vi "颖洁的新生日志_main.vi"() -> ()   [LabVIEW 2011]
panel:
  in  "圈存机":bool
  out "等级":i32=1000
  out "leave":bool
  in  "退出？":bool
  in  "退出游戏":bool
  out "开心值":dbl(slide) scale=0.0..500.0
  out "当前开心值":i32=1000
  out "提示":string
  in  "银行":bool
  out "存款":i32
  in  "云杉轩":bool
  in  "海棠轩":bool
  out "天数":i32
  out "余额":i32
  in  "辛夷阁":bool
  in  "枕雨楼":bool
  in  "库存":i32[](listbox)
  in  "卖出数量":i32 min=0 step=1
  in  "买入数量":i32 min=0 step=1
  in  "卖出":bool
  in  "买入":bool
  in  "商品价格":i32[](listbox)
  out "物品存在索引":i32[](array[numeric])
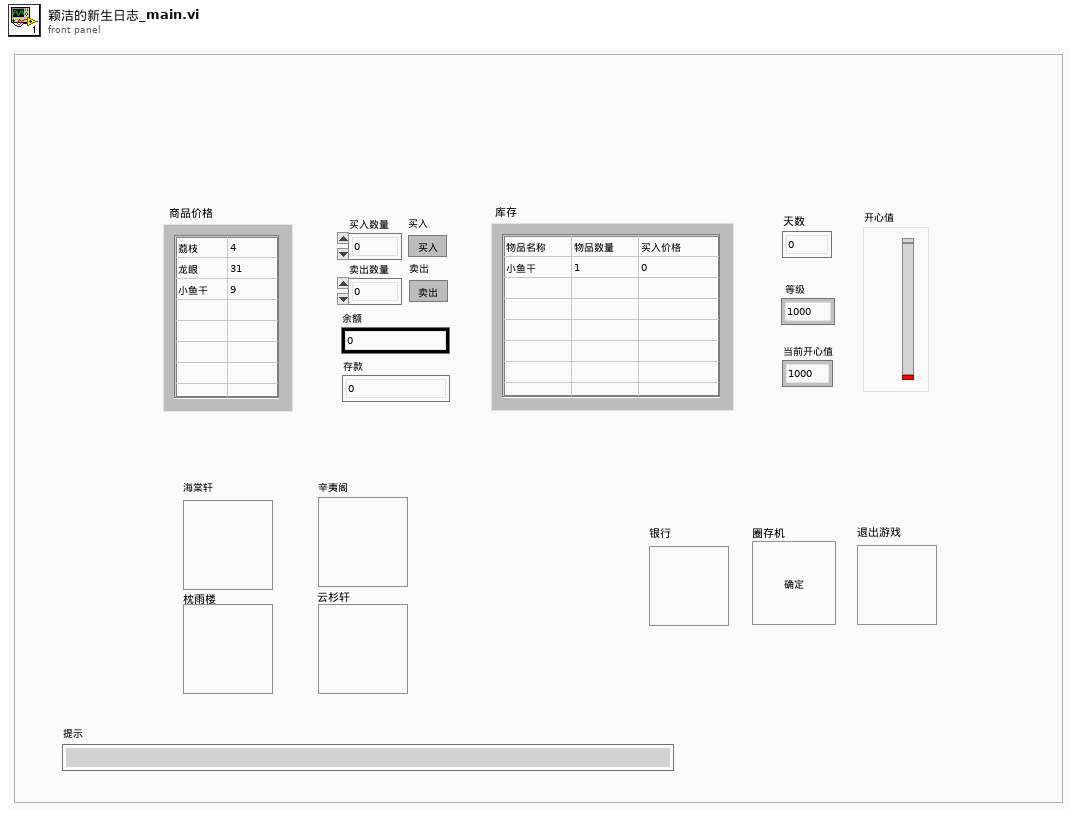
[diagram p1: front panel]
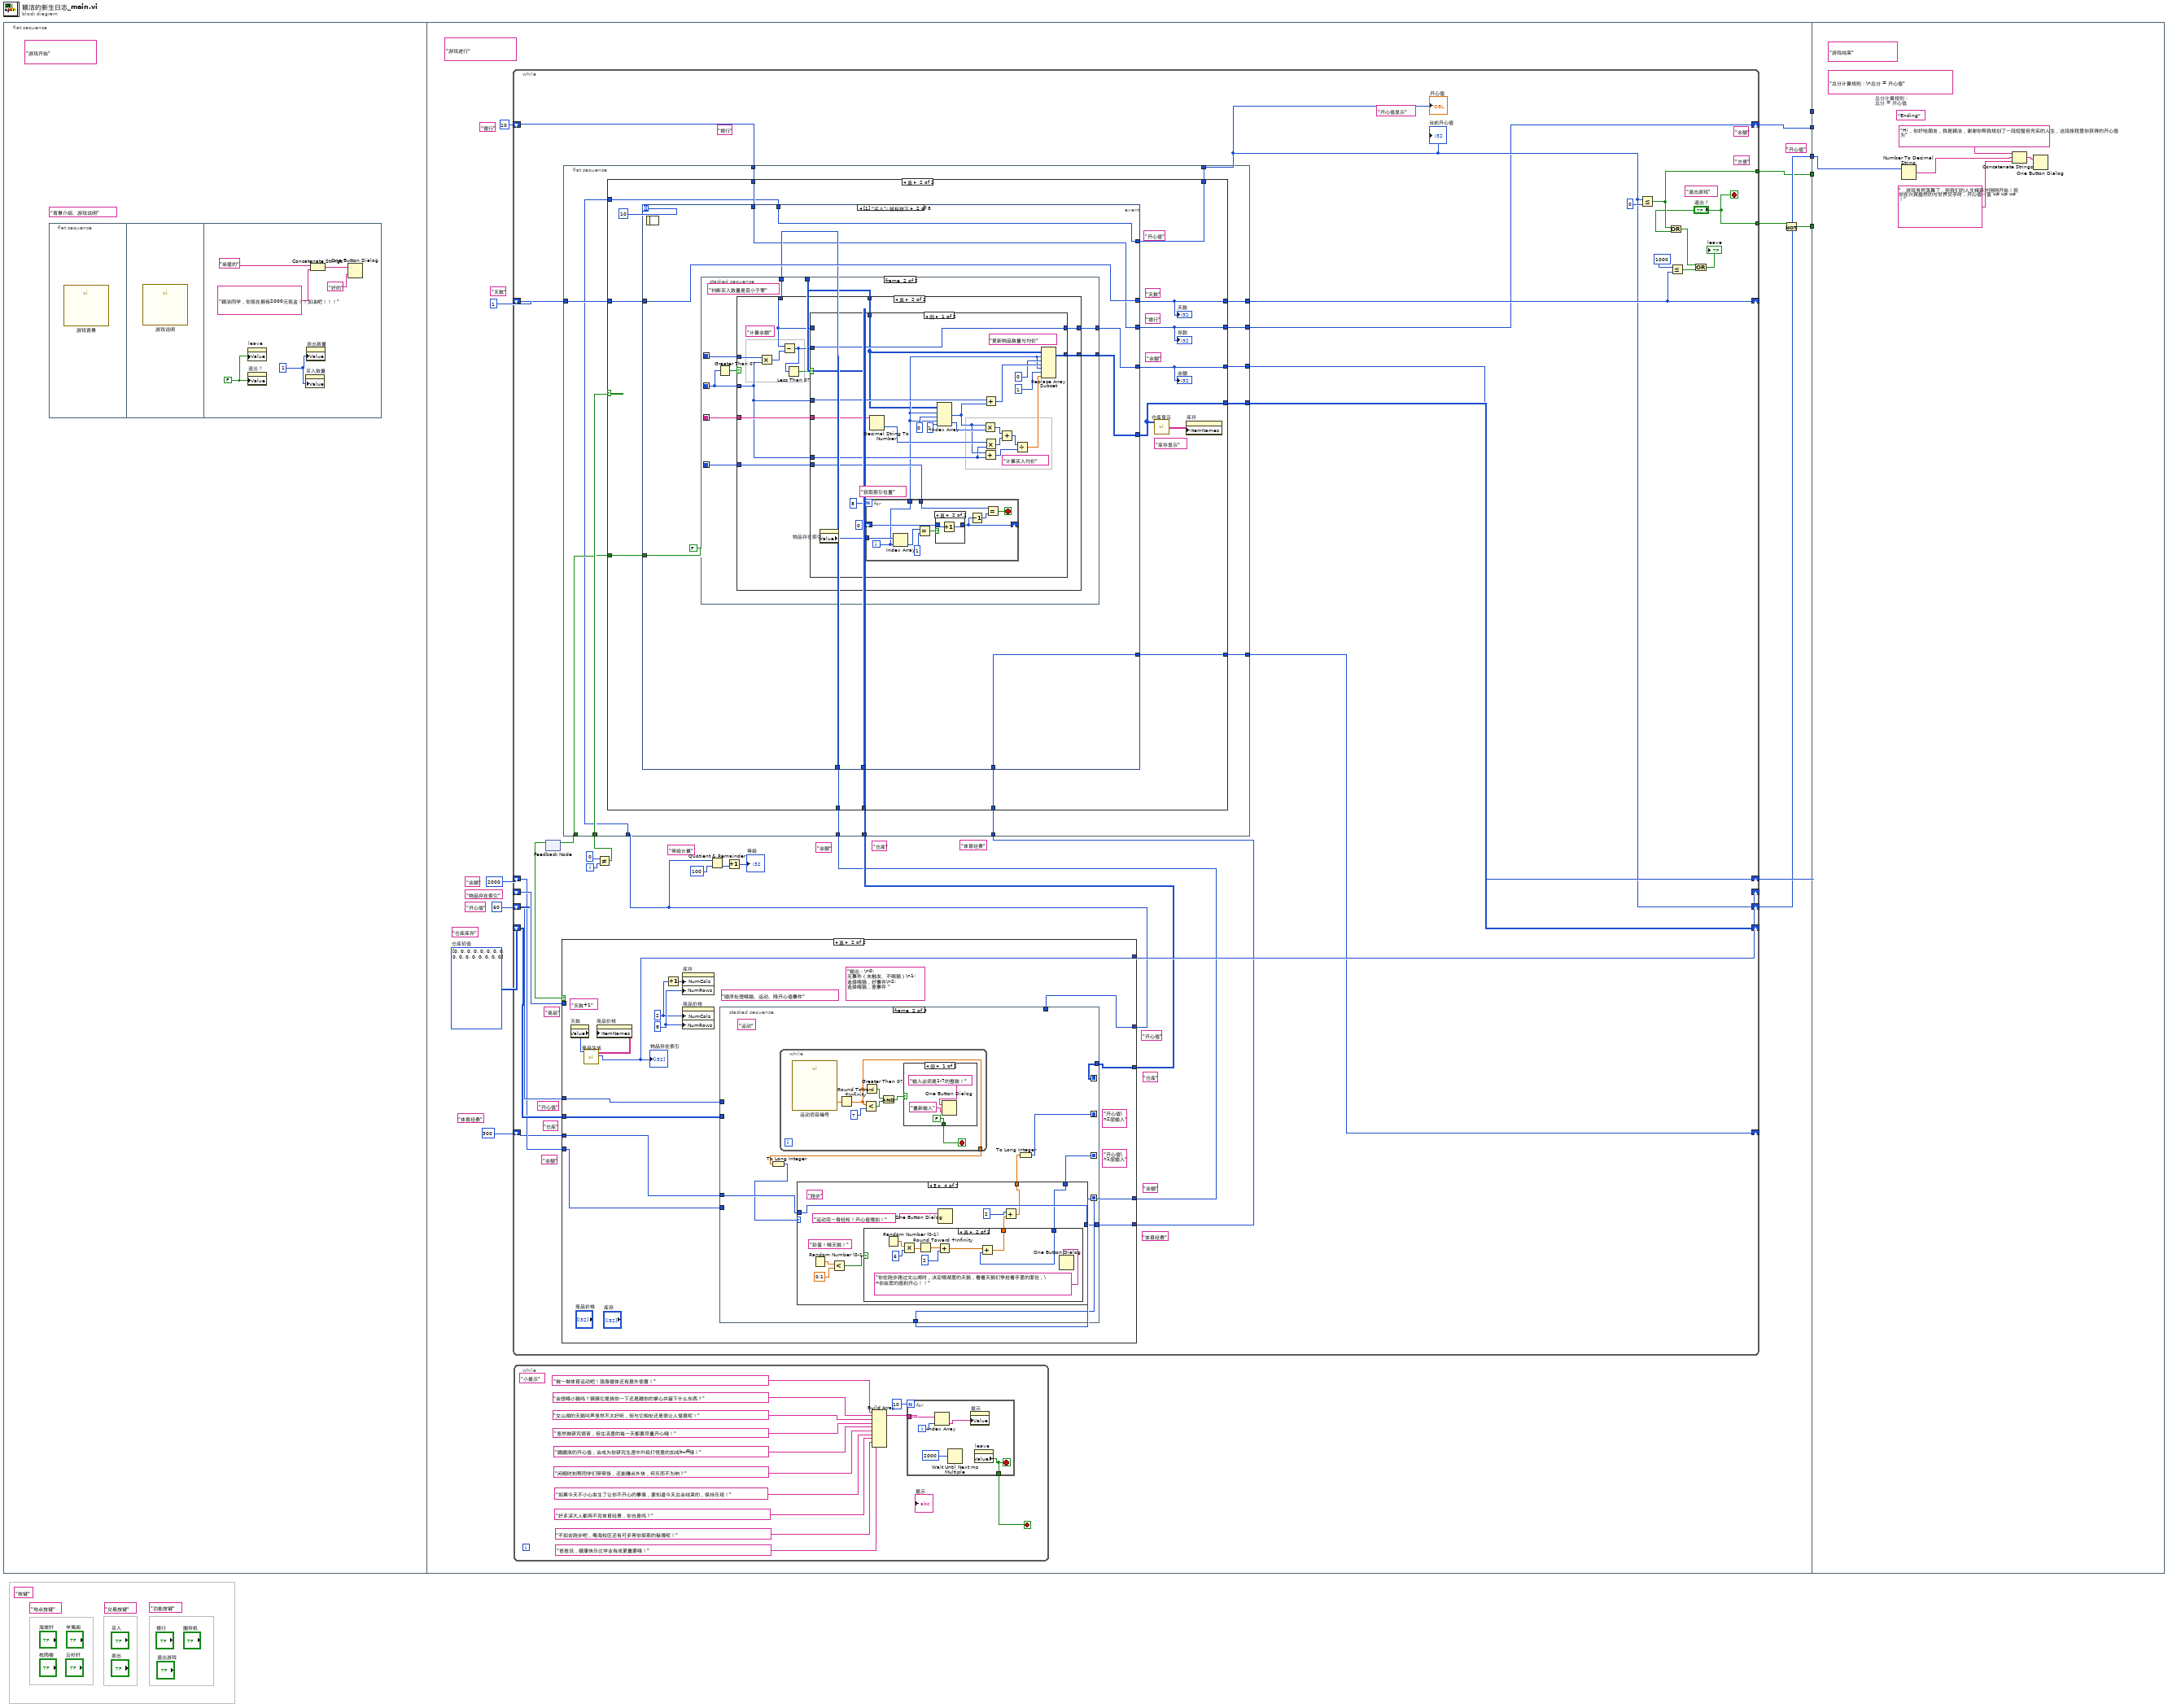
[diagram p0: block diagram]
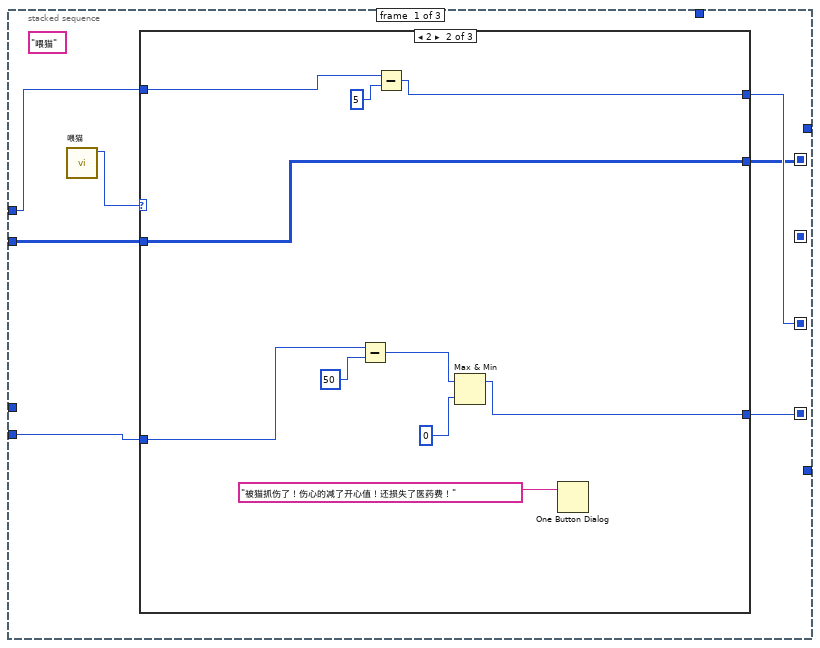
[diagram p3: hidden frame]
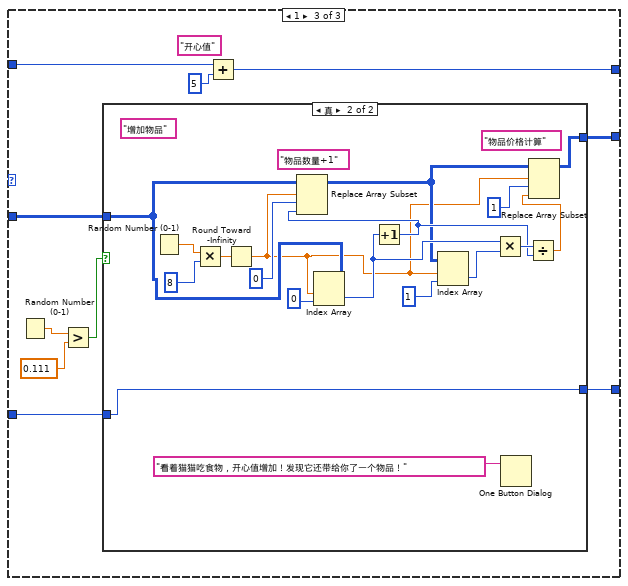
[diagram p5: hidden frame]
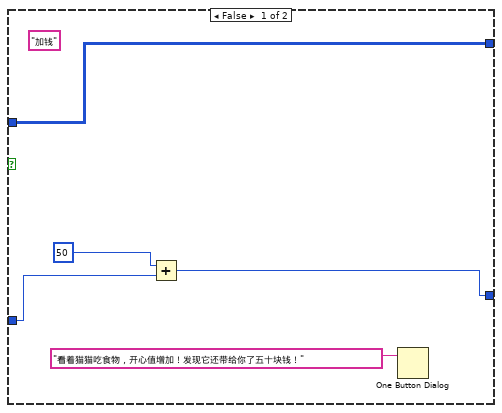
[diagram p6: hidden frame]
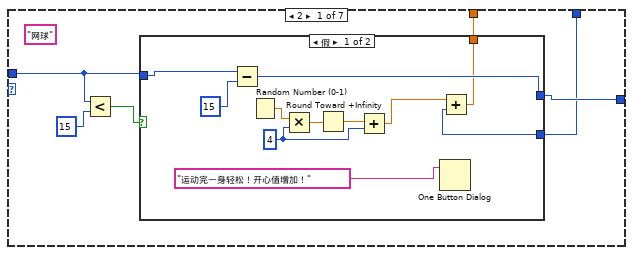
[diagram p7: hidden frame]
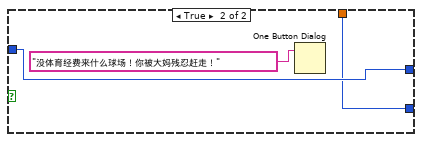
[diagram p8: hidden frame]
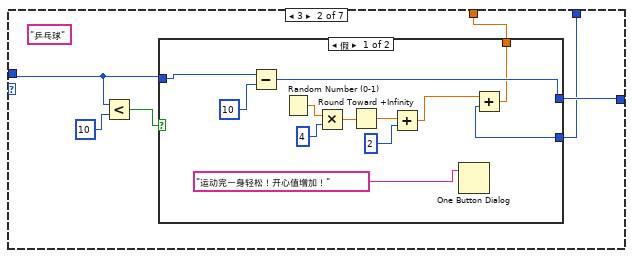
[diagram p9: hidden frame]
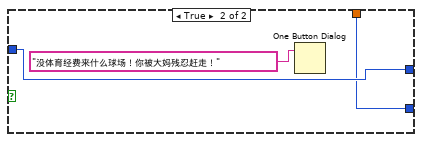
[diagram p10: hidden frame]
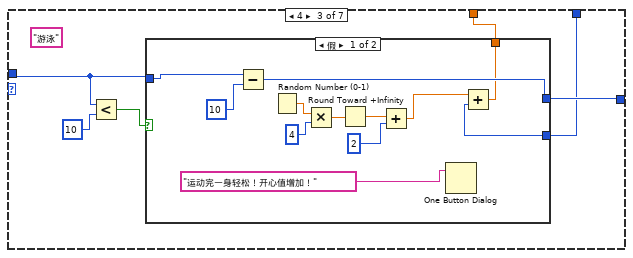
[diagram p11: hidden frame]
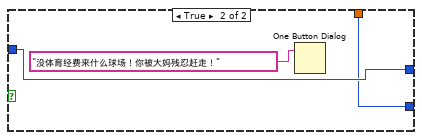
[diagram p12: hidden frame]
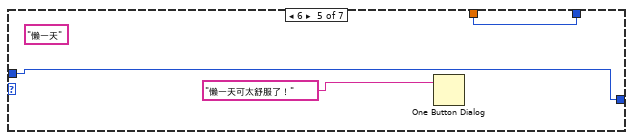
[diagram p14: hidden frame]
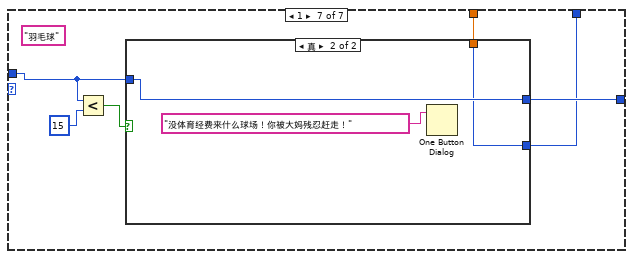
[diagram p16: hidden frame]
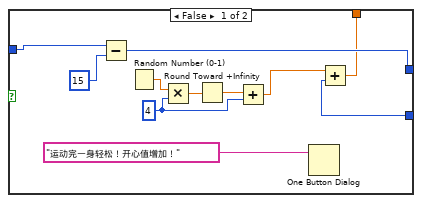
[diagram p17: hidden frame]
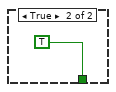
[diagram p18: hidden frame]
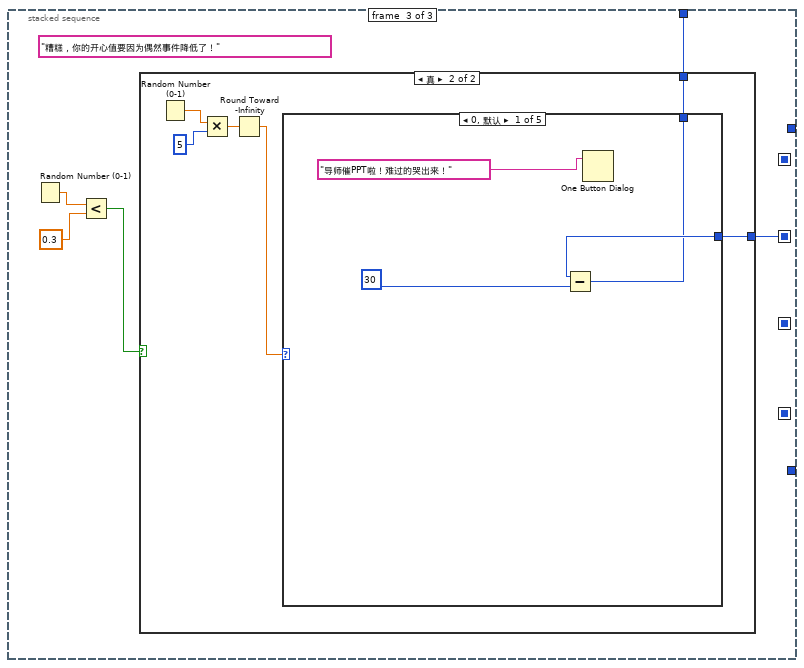
[diagram p19: hidden frame]
diagram:
  (unwired) "功能按键"
  (unwired) "交易按键"
  (unwired) "地点按键"
  (unwired) "按键"
  n1 = flat-sequence {
    tunnel: [w23] -> w5
    tunnel: [w22] -> w4
    tunnel: [w21] -> w3
    tunnel: [w20] -> w2
    tunnel: [w13] -> w1
    tunnel: w5 -> [_]
    tunnel: w4 -> [_]
    tunnel: w3 -> [w659]
    tunnel: w2 -> [_]
    tunnel: w1 -> [_]
    frame #0 {
      (unwired) "背景介绍、游戏说明"
      (unwired) "游戏开始"
      n2 = flat-sequence {
        frame #0 {
          n3 = call "游戏背景"() -> ()  [unwired: 18 in, 2 out]
        }
        frame #1 {
          n4 = call "游戏说明"() -> ()  [unwired: 18 in, 2 out]
        }
        frame #2 {
          w7 = 1
          w8 = FALSE
          n5 = property on="leave" class="Bool (严格)"("Value"=w8) -> ()  [unwired: 2 in, 2 out]
          n6 = property on="退出？" class="Bool (严格)"("Value"=w8) -> ()  [unwired: 2 in, 2 out]
          n7 = property on="买入数量" class="DigNum (严格)"("Value"=w7) -> ()  [unwired: 2 in, 2 out]
          n8 = property on="卖出数量" class="DigNum (严格)"("Value"=w7) -> ()  [unwired: 2 in, 2 out]
          n9 = Concatenate Strings("亲爱的" ("姓名输入提示"), "颖洁同学，你现在拥有2000元现金！！加油吧！！！" ("姓名输入提示")) -> (w10:string)
          n10 = One Button Dialog(message=w10, button name ("OK")="好的" ("姓名输入提示")) -> ()  [unwired: 1 out]
        }
      }
    }
    frame #1 {
      (unwired) "开心值"
      (unwired) "体育经费"
      (unwired) "物品存在索引"
      (unwired) "游戏进行"
      (unwired) "开心值"
      (unwired) "银行"
      (unwired) "仓库库存"
      (unwired) "天数"
      (unwired) "余额"
      w17 = i32[][] [[0, 0], [0, 0], [0, 0], [0, 0], [0, 0], [0, 0], [0, 0], [0, 0]]  # 仓库初值
      n11 = while {
        shift-right: [w69] -> w23
        shift-left: 2000 -> [w52]
        shift-right: [w70] -> _
        shift-left: w17 -> [w54]
        shift-right: [w73] -> _
        shift-left: _ -> [w72]
        shift-right: [w66] -> _
        shift-left: 1 -> [w63]
        shift-right: [w57] -> w22
        shift-left: 10 -> [w64]
        shift-right: [w58] -> w21
        shift-left: 60 -> [w65]
        tunnel: [w59] -> w20
        tunnel: ["退出？"] -> w14
        shift-right: [w44] -> _
        shift-left: 300 -> [w50]
        i -> [w68]
        stop <- "退出？" stop-if-true
        (unwired) "体育经费"
        (unwired) "等级计算"
        (unwired) "仓库"
        (unwired) "体育经费"
        (unwired) "仓库"
        (unwired) "开心值"
        (unwired) "余额"
        (unwired) "余额"
        (unwired) "退出游戏"
        (unwired) "开心值显示"
        (unwired) "开心值"
        (unwired) "余额"
        (unwired) "欠债"
        (unwired) "商品"
        (unwired) "仓库"
        (unwired) "余额"
        (unwired) "银行"
        n12 = feedback-in #1(w56) -> ()
        n13 = feedback #1() -> (w71:bool)  [unwired: 1 in]
        n14 = case shown="真" w71 {
          tunnel: [w79 w89] -> w73
          tunnel: w72 -> [w79 _]
          tunnel: w65 -> [w78 w80]
          tunnel: [w78 w87] -> w49
          tunnel: w54 -> [w77 w86]
          tunnel: [w77 w83] -> w53
          tunnel: w52 -> [w76 w85]
          tunnel: [w76 w84] -> w51
          tunnel: w50 -> [w75 w82]
          tunnel: [w75 w81] -> w45
          frame False {
          }
          frame True {
            (unwired) "开心值\n2层输入"
            (unwired) "开心值\n1层输入"
            (unwired) "输出：\n0: 无事件（未触发、不喂猫）\n1: 选择喂猫，好事件\n2: 选择喂猫，差事件 "
            (unwired) "顺序处理喂猫、运动、降开心值事件"
            (unwired) "天数+1"
            w93 = i8 8
            w91 = i8 2
            n15 = property on="天数" class="DigNum (严格)"() -> ("Value"=w88:i32)  [unwired: 2 in, 2 out]
            n16 = call "商品生成.vi"("天数"=w88) -> ("物品存在索引"=w89:i32[], "市面商品"=w90:string[][])  [unwired: 9 in]
            "物品存在索引" <- w89
            n17 = property on="商品价格" class="MCListbox (严格)"("ItemNames"=w90) -> ()  [unwired: 2 in, 2 out]
            n18 = Increment(x=w91) -> (x+1=w92:i8)
            n19 = property on="库存" class="MCListbox (严格)"("NumCols"=w92, "NumRows"=w93) -> ()  [unwired: 2 in, 2 out]
            n20 = property on="商品价格" class="MCListbox (严格)"("NumCols"=w91, "NumRows"=w93) -> ()  [unwired: 2 in, 2 out]
            n21 = stacked-sequence {
              seq-local: [w99 _ _] -> [_ w152 _]
              seq-local: [w97 _ _] -> [_ w149 _]
              seq-local: [w94 _ _] -> [_ w155 _]
              seq-local: [_ w150 _] -> [_ _ w274]
              tunnel: w80 -> [w100 _ _]
              tunnel: w86 -> [w98 _ _]
              tunnel: w85 -> [w95 _ _]
              tunnel: [_ _ w273] -> w87
              tunnel: [_ w155 _] -> w84
              tunnel: [_ w149 _] -> w83
              tunnel: w82 -> [_ w154 _]
              tunnel: [_ w153 _] -> w81
              frame #0 {
                (unwired) "喂猫"
                n22 = call "喂猫.vi"() -> ("数值"=w96:i8)  [unwired: 11 in]
                n23 = case shown="2" w96 {
                  tunnel: w100 -> [w103 w112 w122]
                  tunnel: [w103 w111 w121] -> w99
                  tunnel: w98 -> [w102 w110 w120]
                  tunnel: [w102 w110 w119] -> w97
                  tunnel: w95 -> [w101 w108 w115]
                  tunnel: [w101 w105 w114] -> w94
                  frame 0, Default {
                  }
                  frame 2 {
                    n24 = Subtract(x=w108, y=50) -> (x-y=w106:i32)
                    n25 = Subtract(x=w112, y=5) -> (x-y=w111:i32)
                    n26 = Max & Min(x=w106, y=0) -> (max(x,y)=w105:i32)  [unwired: 1 out]
                    n27 = One Button Dialog(message="被猫抓伤了！伤心的减了开心值！还损失了医药费！") -> ()  [unwired: 1 in, 1 out]
                  }
                  frame 1 {
                    (unwired) "开心值"
                    n28 = Random Number (0-1)() -> (number: 0 to 1=w118:dbl)
                    n29 = Greater?(x=w118, y=0.111) -> (0:w116:bool)
                    n30 = case shown="真" w116 {
                      tunnel: w120 -> [w128 w141]
                      tunnel: [w128 w131] -> w119
                      tunnel: w115 -> [w127 w130]
                      tunnel: [w125 w130] -> w114
                      frame False {
                        (unwired) "加钱"
                        n31 = Add(x=50, y=w127) -> (x+y=w125:i32)
                        n32 = One Button Dialog(message="看着猫猫吃食物，开心值增加！发现它还带给你了五十块钱！") -> ()  [unwired: 1 in, 1 out]
                      }
                      frame True {
                        (unwired) "物品价格计算"
                        (unwired) "物品数量+1"
                        (unwired) "增加物品"
                        n33 = Random Number (0-1)() -> (number: 0 to 1=w146:dbl)
                        n34 = Multiply(x=w146, y=8) -> (x*y=w144:dbl)
                        n35 = Round Toward -Infinity(1:w144) -> (0:w134:dbl)
                        n36 = Index Array(array=w141, index (row)=w134, index (col)=0) -> (element=w139:i32)
                        n37 = Increment(x=w139) -> (x+1=w136:i32)
                        n38 = Replace Array Subset ("替换数组子集")(array=w141, new element=w136, index (row)=w134, index (col)=0) -> (w135:i32[][])
                        n39 = Index Array(array=w135, index (row)=w134, index (col)=1) -> (element=w142:i32)
                        n40 = Multiply(x=w139, y=w142) -> (x*y=w137:i32)
                        n41 = One Button Dialog(message="看着猫猫吃食物，开心值增加！发现它还带给你了一个物品！") -> ()  [unwired: 1 in, 1 out]
                        n42 = Divide(x=w137, y=w136) -> (x/y=w132:dbl)
                        n43 = Replace Array Subset ("替换数组子集")(array=w135, new element=w132, index (row)=w134, index (col)=1) -> (w131:i32[][])
                      }
                    }
                    n44 = Add(x=w122, y=5) -> (x+y=w121:i32)
                  }
                }
              }
              frame #1 {
                (unwired) "运动"
                n45 = while {
                  tunnel: [w262] -> w148
                  stop <- w263 stop-if-true
                  n46 = call "运动项目编号"() -> ("运动项目"=w268:dbl)  [unwired: 17 in, 2 out]
                  n47 = Round Toward +Infinity(x=w268) -> (ceil(x): smallest int >= x=w262:dbl)
                  n48 = Less?(x=w262, y=7) -> (x < y?=w266:bool)
                  n49 = Greater Than 0?(x=w262) -> (x > 0?=w265:bool)
                  n50 = And(x=w265, y=w266) -> (x .and. y?=w264:bool)
                  n51 = case shown="假" w264 {
                    tunnel: [FALSE TRUE] -> w263
                    frame False {
                      n52 = One Button Dialog(message="输入必须是1-7的整数！", button name ("OK")="重新输入" ("姓名输入提示")) -> ()  [unwired: 1 out]
                    }
                    frame True {
                    }
                  }
                }
                n53 = To Long Integer(number=w148) -> (32bit integer=w147:i32)
                n54 = case shown="5" w147 {
                  tunnel: w154 -> [w158 w178 w199 w226 w238 w240 w244]
                  tunnel: [w159 w179 w200 w226 w238 w240 w245] -> w153
                  tunnel: w152 -> [w157 w177 w198 w221 w237 w241 w243]
                  tunnel: [w156 w176 w197 w218 w237 w241 w242] -> w151
                  frame 2 {
                    (unwired) "网球" ("姓名输入提示")
                    n55 = Less?(x=w158, y=15) -> (x < y?=w160:bool)
                    n56 = case shown="假" w160 {
                      tunnel: w158 -> [w170 w174]
                      tunnel: [w169 w174] -> w159
                      tunnel: w157 -> [w163 w173]
                      tunnel: [w162 w173] -> w156
                      frame False {
                        w165 = 4
                        n57 = Subtract(x=w170, y=15) -> (x-y=w169:i32)
                        n58 = Random Number (0-1)() -> (number: 0 to 1=w168:dbl)
                        n59 = Multiply(x=w168, y=w165) -> (x*y=w167:dbl)
                        n60 = Round Toward +Infinity(x=w167) -> (ceil(x): smallest int >= x=w166:dbl)
                        n61 = Add(x=w166, y=w165) -> (x+y=w164:dbl)
                        n62 = One Button Dialog(message="运动完一身轻松！开心值增加！") -> ()  [unwired: 1 in, 1 out]
                        n63 = Add(x=w164, y=w163) -> (x+y=w162:dbl)
                      }
                      frame True {
                        n64 = One Button Dialog(message="没体育经费来什么球场！你被大妈残忍赶走！") -> ()  [unwired: 1 in, 1 out]
                      }
                    }
                  }
                  frame 3 {
                    (unwired) "乒乓球" ("姓名输入提示")
                    n65 = Less?(x=w178, y=10) -> (x < y?=w181:bool)
                    n66 = case shown="假" w181 {
                      tunnel: w178 -> [w191 w195]
                      tunnel: [w190 w195] -> w179
                      tunnel: w177 -> [w184 w194]
                      tunnel: [w183 w194] -> w176
                      frame False {
                        n67 = Subtract(x=w191, y=10) -> (x-y=w190:i32)
                        n68 = Random Number (0-1)() -> (number: 0 to 1=w189:dbl)
                        n69 = Multiply(x=w189, y=4) -> (x*y=w188:dbl)
                        n70 = Round Toward +Infinity(x=w188) -> (ceil(x): smallest int >= x=w187:dbl)
                        n71 = Add(x=w187, y=2) -> (x+y=w185:dbl)
                        n72 = One Button Dialog(message="运动完一身轻松！开心值增加！") -> ()  [unwired: 1 in, 1 out]
                        n73 = Add(x=w185, y=w184) -> (x+y=w183:dbl)
                      }
                      frame True {
                        n74 = One Button Dialog(message="没体育经费来什么球场！你被大妈残忍赶走！") -> ()  [unwired: 1 in, 1 out]
                      }
                    }
                  }
                  frame 4 {
                    (unwired) "游泳" ("姓名输入提示")
                    n75 = Less?(x=w199, y=10) -> (x < y?=w201:bool)
                    n76 = case shown="假" w201 {
                      tunnel: w199 -> [w212 w216]
                      tunnel: [w211 w216] -> w200
                      tunnel: w198 -> [w205 w215]
                      tunnel: [w204 w215] -> w197
                      frame False {
                        n77 = Subtract(x=w212, y=10) -> (x-y=w211:i32)
                        n78 = Random Number (0-1)() -> (number: 0 to 1=w210:dbl)
                        n79 = Multiply(x=w210, y=4) -> (x*y=w209:dbl)
                        n80 = Round Toward +Infinity(x=w209) -> (ceil(x): smallest int >= x=w208:dbl)
                        n81 = Add(x=w208, y=2) -> (x+y=w206:dbl)
                        n82 = One Button Dialog(message="运动完一身轻松！开心值增加！") -> ()  [unwired: 1 in, 1 out]
                        n83 = Add(x=w206, y=w205) -> (x+y=w204:dbl)
                      }
                      frame True {
                        n84 = One Button Dialog(message="没体育经费来什么球场！你被大妈残忍赶走！") -> ()  [unwired: 1 in, 1 out]
                      }
                    }
                  }
                  frame 5 {
                    (unwired) "彩蛋！喂天鹅！"
                    (unwired) "跑步" ("姓名输入提示")
                    n85 = Random Number (0-1)() -> (number: 0 to 1=w224:dbl)
                    n86 = Less?(x=w224, y=0.1) -> (x < y?=w222:bool)
                    n87 = case shown="真" w222 {
                      tunnel: w221 -> [w227 w229]
                      tunnel: [w227 w228] -> w220
                      frame False {
                      }
                      frame True {
                        n88 = Random Number (0-1)() -> (number: 0 to 1=w235:dbl)
                        n89 = Multiply(x=w235, y=6) -> (x*y=w234:dbl)
                        n90 = Round Toward +Infinity(x=w234) -> (ceil(x): smallest int >= x=w233:dbl)
                        n91 = Add(x=w233, y=2) -> (x+y=w230:dbl)
                        n92 = Add(x=w230, y=w229) -> (x+y=w228:dbl)
                        n93 = One Button Dialog(message="你在跑步路过文山湖时，决定喂湖里的天鹅，看着天鹅们争抢着手里的面包，\n你由衷的感到开心！！") -> ()  [unwired: 1 in, 1 out]
                      }
                    }
                    n94 = One Button Dialog(message="运动完一身轻松！开心值增加！") -> ()  [unwired: 1 in, 1 out]
                    n95 = Add(x=2, y=w220) -> (x+y=w218:dbl)
                  }
                  frame 6 {
                    (unwired) "懒一天" ("姓名输入提示")
                    n96 = One Button Dialog(message="懒一天可太舒服了！") -> ()  [unwired: 1 in, 1 out]
                  }
                  frame 7, Default {
                  }
                  frame 1 {
                    (unwired) "羽毛球" ("姓名输入提示")
                    n97 = Less?(x=w244, y=15) -> (x < y?=w246:bool)
                    n98 = case shown="真" w246 {
                      tunnel: w244 -> [w256 w260]
                      tunnel: [w255 w260] -> w245
                      tunnel: w243 -> [w250 w259]
                      tunnel: [w248 w259] -> w242
                      frame False {
                        w251 = 4
                        n99 = Subtract(x=w256, y=15) -> (x-y=w255:i32)
                        n100 = Random Number (0-1)() -> (number: 0 to 1=w254:dbl)
                        n101 = Multiply(x=w254, y=w251) -> (x*y=w253:dbl)
                        n102 = Round Toward +Infinity(x=w253) -> (ceil(x): smallest int >= x=w252:dbl)
                        n103 = Add(x=w252, y=w251) -> (x+y=w249:dbl)
                        n104 = One Button Dialog(message="运动完一身轻松！开心值增加！") -> ()  [unwired: 1 in, 1 out]
                        n105 = Add(x=w249, y=w250) -> (x+y=w248:dbl)
                      }
                      frame True {
                        n106 = One Button Dialog(message="没体育经费来什么球场！你被大妈残忍赶走！") -> ()  [unwired: 1 in, 1 out]
                      }
                    }
                  }
                }
                n107 = To Long Integer(number=w151) -> (32bit integer=w150:i32)
              }
              frame #2 {
                (unwired) "糟糕，你的开心值要因为偶然事件降低了！"
                n108 = Random Number (0-1)() -> (number: 0 to 1=w277:dbl)
                n109 = Less?(x=w277, y=0.3) -> (x < y?=w275:bool)
                n110 = case shown="真" w275 {
                  tunnel: w274 -> [w278 w280]
                  tunnel: [w278 w279] -> w273
                  frame False {
                  }
                  frame True {
                    n111 = Random Number (0-1)() -> (number: 0 to 1=w283:dbl)
                    n112 = Multiply(x=w283, y=5) -> (x*y=w282:dbl)
                    n113 = Round Toward -Infinity(1:w282) -> (0:w281:dbl)
                    n114 = case shown="0, 默认" w281 {
                      tunnel: w280 -> [w286 w290 w294 w298 w302]
                      tunnel: [w285 w289 w293 w297 w301] -> w279
                      frame 0, Default {
                        n115 = Subtract(x=w286, y=30) -> (x-y=w285:i32)
                        n116 = One Button Dialog(message="导师催PPT啦！难过的哭出来！") -> ()  [unwired: 1 in, 1 out]
                      }
                      frame 1 {
                        n117 = Subtract(x=w290, y=20) -> (x-y=w289:i32)
                        n118 = One Button Dialog(message="今天生病了！开心值下降！") -> ()  [unwired: 1 in, 1 out]
                      }
                      frame 2 {
                        n119 = Subtract(x=w294, y=20) -> (x-y=w293:i32)
                        n120 = One Button Dialog(message="热水器又坏了！！！！") -> ()  [unwired: 1 in, 1 out]
                      }
                      frame 3 {
                        n121 = Subtract(x=w298, y=10) -> (x-y=w297:i32)
                        n122 = One Button Dialog(message="今天要手洗外套啦！") -> ()  [unwired: 1 in, 1 out]
                      }
                      frame 4 {
                        n123 = Subtract(x=w302, y=10) -> (x-y=w301:i32)
                        n124 = One Button Dialog(message="食堂的饭踩雷了！") -> ()  [unwired: 1 in, 1 out]
                      }
                    }
                  }
                }
              }
            }
          }
        }
        n125 = flat-sequence "平铺式顺序结构" {
          tunnel: w51 -> [w318]
          tunnel: [w314] -> w69
          tunnel: w55 -> [w317]
          tunnel: w53 -> [w316]
          tunnel: [w313] -> w70
          tunnel: [w315] -> w56
          tunnel: [w312] -> w66
          tunnel: w64 -> [w310]
          tunnel: [w309] -> w57
          tunnel: [w308] -> w58
          tunnel: w49 -> [w307]
          tunnel: w63 -> [w311]
          tunnel: w45 -> [w306]
          tunnel: [w305] -> w44
          frame #0 {
            n126 = case shown="真" w317 {
              tunnel: w318 -> [w325 w334]
              tunnel: [w325 w330] -> w314
              tunnel: w316 -> [w324 w328]
              tunnel: [w324 w338] -> w313
              tunnel: [TRUE w340] -> w315
              tunnel: [w322 w329] -> w312
              tunnel: w311 -> [w322 w336]
              tunnel: w310 -> [w321 w335]
              tunnel: [w321 w331] -> w309
              tunnel: [w320 w333] -> w308
              tunnel: w307 -> [w320 w332]
              tunnel: w306 -> [w319 w327]
              tunnel: [w319 w326] -> w305
              frame False {
              }
              frame True {
                (unwired) "库存显示"
                (unwired) "余额"
                (unwired) "天数"
                (unwired) "开心值"
                (unwired) "银行"
                n127 = event shown="[1] \"买入\": 鼠标按下" {
                  selector: _ -> [_ _ _ _ _ _ _ _]
                  dyn-events: _ -> [_ _ _ _ _ _ _ _]
                  timeout: 10 -> [_ _ _ _ _ _ _ _]
                  tunnel: [w345 w354 w435 w562 w571 w575 w635 w644] -> w330
                  tunnel: w334 -> [w345 w351 w436 w562 w571 w579 w635 w647]
                  tunnel: [w346 w355 w433 w563 w570 w576 w638 w639] -> w338
                  tunnel: [FALSE FALSE _ TRUE FALSE _ _ _] -> w340
                  tunnel: w328 -> [w346 w356 w434 w563 w570 w576 w638 w639]
                  tunnel: [w344 w352 w431 w558 w568 w574 w634 w641] -> w329
                  tunnel: w336 -> [w344 w352 w431 w560 w568 w574 w634 w641]
                  tunnel: w335 -> [w343 w350 w432 w554 w567 w578 w636 w640]
                  tunnel: [w343 w350 w432 w555 w567 w577 w636 w640] -> w331
                  tunnel: w332 -> [w342 w349 w430 w559 w566 w573 w637 w642]
                  tunnel: [w342 w349 w430 w559 w566 w573 w637 w642] -> w333
                  tunnel: w327 -> [w341 w348 w429 w553 w565 w572 w632 w645]
                  tunnel: [w341 w348 w429 w553 w565 w572 w632 w643] -> w326
                  event Timeout {
                    n128 = event-data() -> ()  [unwired: 1 in, 3 out]
                  }
                  event "买入": Mouse Down {
                    n129 = event-data() -> ()  [unwired: 1 in, 1 out]
                    n130 = stacked-sequence {
                      seq-local: ["买入数量" _] -> [_ w369]
                      seq-local: [w359 _] -> [_ w370]
                      seq-local: [w358 _] -> [_ w366]
                      seq-local: [w357 _] -> [_ w367]
                      tunnel: w351 -> [_ w374]
                      tunnel: w356 -> [_ w373]
                      tunnel: [_ w372] -> w355
                      tunnel: [_ w371] -> w354
                      frame #0 {
                        (unwired) "使用顺序结构，确保物品价格与买入数量为最新参数"
                        (unwired) "买入数量"
                        (unwired) "买入物品价格"
                        n131 = property on="商品价格" class="MCListbox (严格)"() -> ("ItemNames"=w362:string[][], "Value"=w361:i32[])  [unwired: 2 in, 2 out]
                        n132 = Index Array(array=w361, index=0) -> (element=w358:i32)
                        n133 = Index Array(array=w362, index (row)=w358) -> (element=w363:string[])  [unwired: 1 in]
                        n134 = Index Array(array=w363, index=1) -> (element=w357:string)
                        n135 = Decimal String To Number(string=w357) -> (number=w359:i32)  [unwired: 2 in, 1 out]
                      }
                      frame #1 {
                        (unwired) "判断买入数量是否小于零"
                        n136 = Greater Than 0?(x=w369) -> (x > 0?=w368:bool)
                        n137 = case shown="真" w368 {
                          tunnel: w374 -> [w376 w379]
                          tunnel: w367 -> [_ w387]
                          tunnel: w366 -> [_ w386]
                          tunnel: w373 -> [w375 w385]
                          tunnel: [w375 w384] -> w372
                          tunnel: [w376 w383] -> w371
                          tunnel: w370 -> [_ w382]
                          tunnel: w369 -> [_ w378]
                          frame False {
                            n138 = One Button Dialog(message="买入数量不能小于零！！") -> ()  [unwired: 1 in, 1 out]
                          }
                          frame True {
                            (unwired) "计算余额"
                            n139 = Multiply(x=w382, y=w378) -> (x*y=w388:i32)
                            n140 = Subtract(x=w379, y=w388) -> (x-y=w381:i32)
                            n141 = Less Than 0?(x=w381) -> (x < 0?=w380:bool)
                            n142 = case shown="假" w380 {
                              tunnel: [w412 w428] -> w383
                              tunnel: w381 -> [w412 _]
                              tunnel: w379 -> [_ w428]
                              tunnel: w387 -> [w406 _]
                              tunnel: w386 -> [w393 _]
                              tunnel: w385 -> [w389 w427]
                              tunnel: [w399 w427] -> w384
                              tunnel: w378 -> [w395 _]
                              tunnel: w378 -> [w392 _]
                              frame False {
                                (unwired) "更新物品数量与均价"
                                (unwired) "计算买入均价"
                                (unwired) "获取索引位置"
                                n143 = property on="物品存在索引" class="Arr (严格)"() -> ("Value"=w390:i32[])  [unwired: 2 in, 2 out]
                                n144 = for {
                                N: 8 -> [_]
                                tunnel: w390 -> [w422]
                                shift-right: [w418] -> _
                                shift-left: 0 -> [w419]
                                tunnel: w393 -> [w416]
                                tunnel: [w415] -> w391
                                i -> [w415]
                                stop <- w413 stop-if-true
                                n145 = Index Array(array=w422, index=w415) -> (element=w421:i32)
                                n146 = Equal?(x=w421, y=1) -> (x = y?=w414:bool)
                                n147 = case shown="真" w414 {
                                tunnel: w419 -> [w423 w425]
                                tunnel: [w423 w424] -> w418
                                frame False {
                                }
                                frame True {
                                n148 = Increment(x=w425) -> (x+1=w424:i32)
                                }
                                }
                                n149 = Decrement(x=w418) -> (x-1=w417:i32)
                                n150 = Equal?(x=w416, y=w417) -> (x = y?=w413:bool)
                                }
                                n151 = Decimal String To Number(string=w406) -> (number=w405:i32)  [unwired: 2 in, 1 out]
                                n152 = Index Array(array=w389, index (row) #1=w391, index (col) #1=0, index (row) #2=w391, index (col) #2=1) -> (element #1=w402:i32, element #2=w407:i32)
                                n153 = Multiply(x=w402, y=w407) -> (x*y=w404:i32)
                                n154 = Add(x=w402, y=w392) -> (x+y=w400:i32)
                                n155 = Add(x=w395, y=w402) -> (x+y=w409:i32)
                                n156 = Multiply(x=w405, y=w392) -> (x*y=w403:i32)
                                n157 = Add(x=w404, y=w403) -> (x+y=w401:i32)
                                n158 = Divide(x=w401, y=w400) -> (x/y=w396:dbl)
                                n159 = Replace Array Subset(array=w389, new element #1=w409, index (row) #1=w391, index (col) #1=0, new element #2=w396, index (row) #2=w391, index (col) #2=1) -> (w399:i32[][])
                              }
                              frame True {
                                n160 = One Button Dialog(message="余额不足！请重新输入") -> ()  [unwired: 1 in, 1 out]
                              }
                            }
                          }
                        }
                      }
                    }
                  }
                  event "卖出": Mouse Down {
                    n161 = event-data() -> ()  [unwired: 1 in, 1 out]
                    n162 = stacked-sequence {
                      seq-local: ["卖出数量" _] -> [_ w446]
                      seq-local: [w442 _] -> [_ w454]
                      seq-local: [w437 _] -> [_ w450]
                      tunnel: w434 -> [_ w453]
                      tunnel: w436 -> [_ w452]
                      tunnel: [_ w451] -> w435
                      tunnel: [_ w449] -> w433
                      tunnel: w430 -> [_ w448]
                      frame #0 {
                        n163 = property on="库存" class="MCListbox (严格)"() -> ("ItemNames"=w440:string[][], "Value"=w439:i32[])  [unwired: 2 in, 2 out]
                        n164 = Index Array(array=w439, index=0) -> (element=w437:i32)
                        n165 = Index Array(array=w440, index (row)=w437) -> (element=w441:string[])  [unwired: 1 in]
                        n166 = Index Array(array=w441, index=1) -> (element=w443:string)
                        n167 = Decimal String To Number(string=w443) -> (number=w442:i32)  [unwired: 2 in, 1 out]
                      }
                      frame #1 {
                        (unwired) "库存\n索引"
                        (unwired) "库存\n数量"
                        (unwired) "卖出\n数量"
                        (unwired) "判断卖出数量是否大于零"
                        n168 = Greater Or Equal To 0?(x=w446) -> (x >= 0?=w447:bool)
                        n169 = case shown="真" w447 {
                          tunnel: w454 -> [_ w467]
                          tunnel: w453 -> [w455 w465]
                          tunnel: w452 -> [w456 w464]
                          tunnel: [w456 w463] -> w451
                          tunnel: w450 -> [_ w462]
                          tunnel: w446 -> [_ w460]
                          tunnel: [w455 w459] -> w449
                          tunnel: w448 -> [_ w458]
                          frame False {
                            n170 = One Button Dialog(message="卖出数量不能为负数！！！") -> ()  [unwired: 1 in, 1 out]
                          }
                          frame True {
                            (unwired) "判断是否选中商品"
                            n171 = Less?(x=w467, y=w460) -> (x < y?=w466:bool)
                            n172 = Not Equal To 0?(x=w462) -> (x != 0?=w461:bool)
                            n173 = case shown="真" w461 {
                              tunnel: w466 -> [_ w474]
                              tunnel: w465 -> [w468 w478]
                              tunnel: w462 -> [_ w477]
                              tunnel: w460 -> [_ w476]
                              tunnel: w464 -> [w469 w471]
                              tunnel: [w469 w475] -> w463
                              tunnel: [w468 w473] -> w459
                              tunnel: w458 -> [_ w472]
                              frame False {
                                n174 = One Button Dialog(message="没有选中商品！请重新选择~") -> ()  [unwired: 1 in, 1 out]
                              }
                              frame True {
                                (unwired) "判断卖出数量是否超过库存量"
                                n175 = case shown="假" w474 {
                                tunnel: w478 -> [w484 w551]
                                tunnel: w477 -> [w489 _]
                                tunnel: w476 -> [w479 _]
                                tunnel: [w485 w550] -> w475
                                tunnel: [w482 w551] -> w473
                                tunnel: w472 -> [w481 _]
                                tunnel: w471 -> [w480 w550]
                                frame False {
                                (unwired) "判断市面中是否存在卖出商品"
                                (unwired) "索引所选择商品"
                                n176 = for {
                                N: 8 -> [_]
                                tunnel: w484 -> [w542]
                                shift-right: [w544] -> _
                                shift-left: 0 -> [w540]
                                tunnel: w489 -> [w541]
                                tunnel: [w539] -> w483
                                i -> [w539]
                                stop <- w543 stop-if-true
                                n177 = Index Array(array=w542, index (row)=w539, index (col)=0) -> (element=w546:i32)
                                n178 = Not Equal To 0?(x=w546) -> (x != 0?=w545:bool)
                                n179 = case shown="真" w545 {
                                tunnel: [w547 w549] -> w544
                                tunnel: w540 -> [w547 w548]
                                frame False {
                                }
                                frame True {
                                n180 = Increment(x=w548) -> (x+1=w549:i32)
                                }
                                }
                                n181 = Equal?(x=w544, y=w541) -> (x = y?=w543:bool)
                                }
                                n182 = property on="物品存在索引" class="Arr (严格)"() -> ("Value"=w486:i32[])  [unwired: 2 in, 2 out]
                                n183 = Index Array(array=w486, index=w483) -> (element=w488:i32)
                                n184 = Not Equal To 0?(x=w488) -> (x != 0?=w487:bool)
                                n185 = case shown="真" w487 {
                                tunnel: w483 -> [_ w525]
                                tunnel: w486 -> [_ w526]
                                tunnel: w479 -> [_ w506]
                                tunnel: w480 -> [w493 w520]
                                tunnel: [w493 w519] -> w485
                                tunnel: w484 -> [_ w517]
                                tunnel: w483 -> [_ w516]
                                tunnel: w479 -> [_ w514]
                                tunnel: w484 -> [w492 w511]
                                tunnel: w483 -> [_ w510]
                                tunnel: [w492 w509] -> w482
                                tunnel: w481 -> [_ w505]
                                frame False {
                                n186 = One Button Dialog(message="黑市并没有该商品的交易！先屯着吧~") -> ()  [unwired: 1 in, 1 out]
                                }
                                frame True {
                                (unwired) "判断库存是否卖完"
                                (unwired) "去除库存"
                                (unwired) "余额计算"
                                n187 = property on="商品价格" class="MCListbox (严格)"() -> ("ItemNames"=w523:string[][])  [unwired: 2 in, 2 out]
                                n188 = Array Subset(array=w526, length=w525) -> (w524:i32[])  [unwired: 1 in]
                                n189 = Index Array(array=w517, index (row)=w516, index (col)=0) -> (element=w513:i32)
                                n190 = Add Array Elements(numeric array=w524) -> (sum=w522:i32)
                                n191 = Subtract(x=w513, y=w514) -> (x-y=w508:i32)
                                n192 = Equal To 0?(x=w508) -> (x = 0?=w512:bool)
                                n193 = Index Array(array=w523, index (row)=w522, index (col)=1) -> (element=w507:string)
                                n194 = case shown="假" w512 {
                                tunnel: w511 -> [w532 w537]
                                tunnel: w510 -> [w531 w536]
                                tunnel: [w528 w533] -> w509
                                tunnel: w508 -> [w529 _]
                                frame False {
                                n195 = Replace Array Subset(array=w532, new element=w529, index (row)=w531, index (col)=0) -> (w528:i32[][])
                                }
                                frame True {
                                w534 = 0
                                n196 = Increment(x=w534) -> (x+1=w535:i32)
                                n197 = Replace Array Subset(array=w537, new element #1=w534, index (row) #1=w536, index (col) #1=w534, new element #2=w534, index (row) #2=w536, index (col) #2=w535) -> (w533:i32[][])
                                }
                                }
                                n198 = Decimal String To Number(string=w507) -> (number=w518:i32)  [unwired: 2 in, 1 out]
                                n199 = Multiply(x=w518, y=w506) -> (x*y=w499:i32)
                                n200 = Quotient & Remainder(x=w505, y=100) -> (floor(x/y)=w496:i32)  [unwired: 1 out]
                                n201 = Decrement(x=w496) -> (x-1=w498:i32)
                                n202 = Greater Than 0?(x=w498) -> (x > 0?=w497:bool)
                                n203 = Multiply(x=w496, y=0.1) -> (x*y=w501:dbl)
                                n204 = case shown="真" w497 {
                                frame False {
                                }
                                frame True {
                                n205 = One Button Dialog(message="满满的开心值让你在与买家的谈判中游刃有余，卖出价格超过市面价格！") -> ()  [unwired: 1 in, 1 out]
                                }
                                }
                                n206 = Increment(x=w501) -> (x+1=w495:dbl)
                                n207 = Multiply(x=w495, y=w499) -> (x*y=w500:dbl)
                                n208 = To Long Integer(number=w500) -> (32bit integer=w502:i32)
                                n209 = Add(x=w502, y=w520) -> (x+y=w519:i32)
                                }
                                }
                                }
                                frame True {
                                n210 = One Button Dialog(message="库存太少啦！请重新选择~") -> ()  [unwired: 1 in, 1 out]
                                }
                                }
                              }
                            }
                          }
                        }
                      }
                    }
                  }
                  event "枕雨楼", "海棠轩", "云杉轩", "辛夷阁": Mouse Up {
                    n211 = event-data() -> ()  [unwired: 1 in, 8 out]
                    n212 = Add(x=1, y=w560) -> (x+y=w558:i32)
                    n213 = Multiply(x=w554, y=1.05) -> (x*y=w556:dbl)
                    n214 = To Long Integer(number=w556) -> (32bit integer=w555:i32)
                  }
                  event "库存", "商品价格": Mouse Down {
                    n215 = event-data() -> ()  [unwired: 1 in, 8 out]
                  }
                  event "银行": Mouse Down {
                    n216 = event-data() -> ()  [unwired: 1 in, 1 out]
                    n217 = Two Button Dialog(message="欢迎来到 IronBank ，你打算干什么？", 1:"取款", 2:"存款") -> (T button?=w580:bool)
                    n218 = case shown="真" w580 {
                      tunnel: w579 -> [w590 w614]
                      tunnel: w578 -> [w589 w613]
                      tunnel: [w588 w612] -> w575
                      tunnel: [w587 w611] -> w577
                      frame False {
                        (unwired) "取款"
                        n219 = call "输入取款数额"() -> ("取款数额"=w585:dbl)  [unwired: 17 in, 2 out]
                        n220 = To Long Integer(number=w585) -> (32bit integer=w584:i32)
                        n221 = Greater Or Equal To 0?(x=w584) -> (x >= 0?=w586:bool)
                        n222 = case shown="真" w586 {
                          tunnel: w590 -> [w593 w598]
                          tunnel: w589 -> [w592 w595]
                          tunnel: [w592 w597] -> w588
                          tunnel: [w593 w596] -> w587
                          tunnel: w584 -> [_ w594]
                          frame False {
                            n223 = One Button Dialog(message="取款数额必须大于等于0！") -> ()  [unwired: 1 in, 1 out]
                          }
                          frame True {
                            n224 = Less?(x=w595, y=w594) -> (x < y?=w599:bool)
                            n225 = case shown="假" w599 {
                              tunnel: [w604 w605] -> w597
                              tunnel: [w603 w606] -> w596
                              tunnel: w594 -> [w602 _]
                              tunnel: w598 -> [w601 w605]
                              tunnel: w595 -> [w600 w606]
                              frame False {
                                n226 = Subtract(x=w600, y=w602) -> (x-y=w603:i32)
                                n227 = Add(x=w601, y=w602) -> (x+y=w604:i32)
                              }
                              frame True {
                                n228 = One Button Dialog(message="余额不足！请重新输入") -> ()  [unwired: 1 in, 1 out]
                              }
                            }
                          }
                        }
                      }
                      frame True {
                        (unwired) "存款"
                        n229 = call "输入存款数额"() -> ("存款数额"=w609:dbl)  [unwired: 17 in, 2 out]
                        n230 = To Long Integer(number=w609) -> (32bit integer=w608:i32)
                        n231 = Greater Or Equal To 0?(x=w608) -> (x >= 0?=w610:bool)
                        n232 = case shown="真" w610 {
                          tunnel: w614 -> [w615 w622]
                          tunnel: w613 -> [w616 w621]
                          tunnel: [w615 w620] -> w612
                          tunnel: [w616 w619] -> w611
                          tunnel: w608 -> [_ w618]
                          frame False {
                            n233 = One Button Dialog(message="存款数额必须大于等于0！") -> ()  [unwired: 1 in, 1 out]
                          }
                          frame True {
                            n234 = Less?(x=w622, y=w618) -> (x < y?=w623:bool)
                            n235 = case shown="假" w623 {
                              tunnel: w618 -> [w628 _]
                              tunnel: [w627 w630] -> w620
                              tunnel: [w626 w629] -> w619
                              tunnel: w622 -> [w625 w630]
                              tunnel: w621 -> [w624 w629]
                              frame False {
                                n236 = Add(x=w624, y=w628) -> (x+y=w626:i32)
                                n237 = Subtract(x=w625, y=w628) -> (x-y=w627:i32)
                              }
                              frame True {
                                n238 = One Button Dialog(message="余额不足！请重新输入") -> ()  [unwired: 1 in, 1 out]
                              }
                            }
                          }
                        }
                      }
                    }
                  }
                  event "退出游戏": Mouse Down {
                    n239 = event-data() -> ()  [unwired: 1 in, 1 out]
                    n240 = property on="退出？" class="Bool (严格)"("Value"=TRUE) -> ()  [unwired: 2 in, 2 out]
                  }
                  event "圈存机": Mouse Down {
                    n241 = event-data() -> ()  [unwired: 1 in, 8 out]
                    n242 = call "输入充值数额"() -> ("充值数额"=w649:dbl)  [unwired: 17 in, 2 out]
                    n243 = To Long Integer(number=w649) -> (32bit integer=w646:i32)
                    n244 = Greater?(x=w646, y=w647) -> (0:w648:bool)
                    n245 = case shown="真" w648 {
                      tunnel: w647 -> [w654 w657]
                      tunnel: w646 -> [w652 _]
                      tunnel: w645 -> [w653 w656]
                      tunnel: [w651 w657] -> w644
                      tunnel: [w650 w656] -> w643
                      frame False {
                        n246 = Subtract(x=w654, y=w652) -> (x-y=w651:i32)
                        n247 = Add(x=w653, y=w652) -> (x+y=w650:i32)
                        n248 = One Button Dialog(message="充值成功！") -> ()  [unwired: 1 in, 1 out]
                      }
                      frame True {
                        n249 = One Button Dialog(message="余额不足！充值失败！") -> ()  [unwired: 1 in, 1 out]
                      }
                    }
                  }
                }
                "余额" <- w330
                "天数" <- w329
                "存款" <- w331
                n250 = call "仓库显示.vi"("仓库"=w338) -> ("显示栏"=w337:string[][])  [unwired: 10 in]
                n251 = property on="库存" class="MCListbox (严格)"("ItemNames"=w337) -> ()  [unwired: 2 in, 2 out]
              }
            }
          }
        }
        n252 = Not Equal?(x=0, y=w68) -> (x != y?=w55:bool)
        n253 = Quotient & Remainder(x=w49, y=100) -> (floor(x/y)=w47:i32)  [unwired: 1 out]
        n254 = Increment(x=w47) -> (x+1=→"等级":i32)
        n255 = Less Or Equal?(x=w58, y=0) -> (x <= y?=w59:bool)
        n256 = Or(x=w59, y="退出？") -> (x .or. y?=w60:bool)
        n257 = Less Or Equal?(x=1000, y=w66) -> (x <= y?=w62:bool)
        n258 = Or(x=w60, y=w62) -> (x .or. y?=→"leave":bool)
        "当前开心值" <- w58
        "开心值" <- w58
      }
      n259 = while {
        stop <- w34 stop-if-true
        (unwired) "小提示"
        n260 = Build Array("做一做体育运动吧！强身健体还有意外惊喜！", "会想喂小猫吗？猜猜它是挠你一下还是蹭你的掌心并留下什么东西？", "文山湖的天鹅叫声虽然不太好听，但与它相处还是很让人惬意呢！", "虽然做研究很苦，但生活里的每一天都要尽量开心哦！", "蹭蹭涨的开心值，会成为你研究生涯中升级打怪里的加成buff哦！", "闲暇时刻帮同学们带带饭，还能赚点外快，何乐而不为呐？", "如果今天不小心发生了让你不开心的事情，要知道今天总会结束的，保持乐观！", "好多深大人都用不完体育经费，你也是吗？", "不如去跑步吧，粤海校区还有可多等你探索的秘境呢！", "爸爸说，健康快乐比学业有成更重要哦！") -> (w36:string[])
        n261 = for {
          N: 10 -> [_]
          tunnel: w36 -> [w41]
          tunnel: [w38] -> w34
          i -> [w40]
          stop <- w38 stop-if-true
          n262 = Index Array(array=w41, index=w40) -> (element=w37:string)
          n263 = Wait Until Next ms Multiple(millisecond multiple=2000) -> ()  [unwired: 1 out]
          n264 = property on="提示" class="Str"("Value"=w37) -> ()  [unwired: 2 in, 2 out]
          n265 = property on="leave" class="Bool (严格)"() -> ("Value"=w38:bool)  [unwired: 2 in, 2 out]
        }
      }
      n266 = Not(x=w14) -> (.not. x?=w13:bool)
    }
    frame #2 {
      (unwired) "Ending"
      (unwired) "总分计算规则：\n总分 = 开心值"  # 总分计算规则： 总分 = 开心值
      (unwired) "游戏结束"
      n267 = Number To Decimal String(number=w659) -> (decimal integer string=w661:string)  [unwired: 1 in]
      n268 = Concatenate Strings("Hi，你好哇朋友，我是颖洁，谢谢你帮我规划了一段短暂但充实的人生，这段旅程里你获得的开心值为", w661, "，游戏虽然落幕了，但我们的人生精彩才刚刚开始！祝你在兴致盎然的与世界交手时，开心值一直 up up up ！") -> (w662:string)
      n269 = One Button Dialog(message=w662) -> ()  [unwired: 1 in, 1 out]
    }
  }
